vi "test Import-Export Custom Device.vi"(8 "error in":errorcluster, 11 "TestCase in":refnum<class "Scripting.lvclass">) -> (0 "error out":errorcluster, 3 "TestCase out":refnum<class "Scripting.lvclass">)   [LabVIEW 2020, in "Scripting.lvclass"]
uses:
  Scripting.lvclass
  C:/dev/git/niveristand-custom-device-testing-tools/VeriStandScriptingTestCase/VeriStandScriptingTestCase.lvclass
  niveristand-custom-device-testing-tools/VeriStandScriptingTestCase/VeriStandScriptingTestCase.lvclass/VeriStandScriptingTestCase.ctl
  NationalInstruments.VeriStand.SystemDefinitionAPI
  niveristand-custom-device-testing-tools/VeriStandScriptingTestCase/Read Target.vi
  Scripting/Custom Device/Import Custom Device (In Place).vi
  Scripting/Custom Device/Import Custom Device (New).vi
  Scripting/AIM MIL-STD-1553 Scripting.lvlib
  <vilib>/addons/_JKI Toolkits/VI Tester/TestCase.llb/TestCase.lvclass
  niveristand-custom-device-testing-tools/VeriStandTestUtilities/VeriStandTestUtilities.lvlib
  C:/Program Files (x86)/National Instruments/LabVIEW 2020/vi.lib/addons/_JKI Toolkits/VI Tester/TestCase.llb/TestCase.lvclass
  C:/dev/git/niveristand-aim-milStd1553-custom-device/Source/Custom Device Support/Tests/Unit/Scripting/Scripting.lvclass
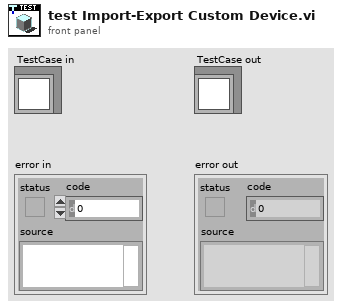
[diagram p1: front panel]
types:
  T1 = typedef "Custom Device API.lvlib/Custom Device Item Ref.ctl" = u64
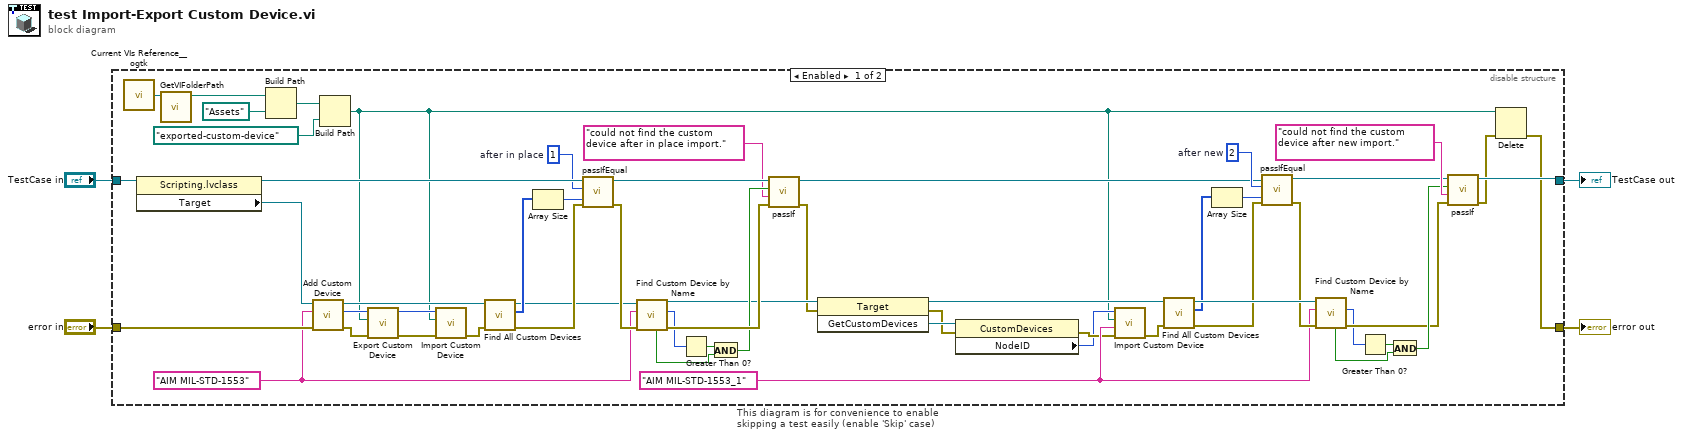
[diagram p0: block diagram]
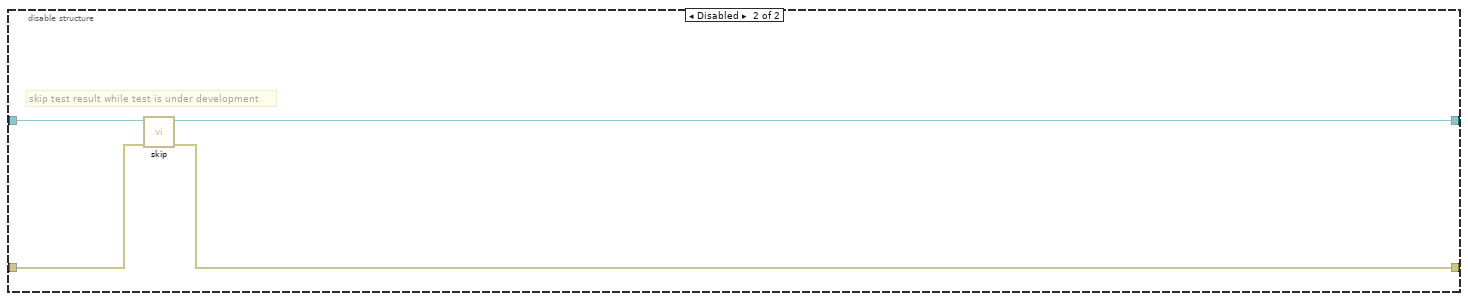
[diagram p2: hidden frame]
diagram:
  n1 = disable-structure "This diagram is for convenience to enable skipping a test easily (enable 'Skip' case)" shown="Enabled" {
    disable-tunnel: "TestCase in" -> [w59 w64]
    disable-tunnel: [w16 w62] -> w4
    disable-tunnel: [w5 w63] -> w2
    disable-tunnel: "error in" -> [w60 w61]
    frame Enabled {
      w17 = "AIM MIL-STD-1553_1" ("name")
      w22 = 2  # after new
      w43 = 1  # after in place
      w39 = "AIM MIL-STD-1553" ("name")
      n2 = call <userlib>:"Current VIs Reference__ogtk.vi"() -> ("Current VI's reference"=w52:refnum<vi>)  [unwired: 5 in]
      n3 = property class="Scripting.lvclass"(reference=w59) -> (reference out=w57:refnum<class "Scripting.lvclass">, "Target"=w58:refnum<k24>)  [unwired: 1 in, 1 out]
      n4 = call "GetVIFolderPath.vi"("VI Reference in"=w52) -> ("VI Folder Path out"=w51:path)  [unwired: 9 in, 1 out]
      n5 = Build Path(base path=w51, name or relative path=path "Assets") -> (appended path=w49:path)
      n6 = call "Add Custom Device.vi"("error in"=w60, "custom device name"=w39, "target"=w58) -> ("error out"=w54:errorcluster, "custom device"=w55:T1, "target out"=w47:refnum<k24>)  [unwired: 6 in]
      n7 = Build Path(base path=w49, name or relative path=path "exported-custom-device") -> (appended path=w7:path)
      n8 = call "Export Custom Device.vi"("error in"=w54, "path"=w7, "custom device"=w55) -> ("error out"=w53:errorcluster, "custom device out"=w56:T1)  [unwired: 7 in]
      n9 = call-poly "Import Custom Device.vi"("error in"=w53, "path"=w7, "custom device"=w56) -> ("error out"=w46:errorcluster)  [unwired: 7 in, 1 out]
      n10 = call "Find All Custom Devices.vi"("error in"=w46, "target"=w47) -> ("error out"=w42:errorcluster, "custom devices"=w45:T1[], "target out"=w40:refnum<k24>)  [unwired: 7 in]
      n11 = Array Size(array=w45) -> (size(s)=w44:i32)
      n12 = call-dynamic "passIfEqual.vi"("error in (no error)"=w42, "y"=w44, "x"=w43, "TestCase in"=w57) -> ("error out"=w41:errorcluster, "TestCase out"=w36:refnum<class "Scripting.lvclass">)  [unwired: 6 in]
      n13 = call "Find Custom Device by Name.vi"("error in"=w41, "custom device name"=w39, "target"=w40) -> ("error out"=w35:errorcluster, "custom device"=w15:T1, "target out"=w12:refnum<k24>, "found?"=w37:bool)  [unwired: 5 in]
      n14 = Greater Than 0?(x=w15) -> (x > 0?=w38:bool)
      n15 = And(x=w38, y=w37) -> (x .and. y?=w34:bool)
      n16 = call-dynamic "passIf.vi"("error in (no error)"=w35, "message (\"\")"="could not find the custom device after in place import." ("message (\"\")"), "pass"=w34, "TestCase in"=w36) -> ("error out"=w9:errorcluster, "TestCase out"=w18:refnum<class "Scripting.lvclass">)  [unwired: 6 in]
      n17 = invoke on="Invoke Node" class="Target" method="GetCustomDevices"(reference=w12, error in=w9) -> (reference out=w11:refnum<k24>, error out=w13:errorcluster, "GetCustomDevices"=w14:refnum<k24>)  [unwired: 1 in]
      n18 = property on="Property Node" class="CustomDevices"(reference=w14, error in=w13) -> (error out=w10:errorcluster, "NodeID"=w8:u64)  [unwired: 1 out]
      n19 = call-poly "Import Custom Device.vi"("error in"=w10, "name"=w17, "path"=w7, "custom devices"=w8) -> ("error out"=w19:errorcluster)  [unwired: 5 in, 2 out]
      n20 = call "Find All Custom Devices.vi"("error in"=w19, "target"=w11) -> ("error out"=w23:errorcluster, "custom devices"=w20:T1[], "target out"=w25:refnum<k24>)  [unwired: 7 in]
      n21 = Array Size(array=w20) -> (size(s)=w21:i32)
      n22 = call-dynamic "passIfEqual.vi"("error in (no error)"=w23, "y"=w21, "x"=w22, "TestCase in"=w18) -> ("error out"=w24:errorcluster, "TestCase out"=w29:refnum<class "Scripting.lvclass">)  [unwired: 6 in]
      n23 = call "Find Custom Device by Name.vi"("error in"=w24, "custom device name"=w17, "target"=w25) -> ("error out"=w30:errorcluster, "custom device"=w26:T1, "found?"=w28:bool)  [unwired: 5 in, 1 out]
      n24 = Greater Than 0?(x=w26) -> (x > 0?=w27:bool)
      n25 = And(x=w27, y=w28) -> (x .and. y?=w31:bool)
      n26 = call-dynamic "passIf.vi"("error in (no error)"=w30, "message (\"\")"="could not find the custom device after new import." ("message (\"\")"), "pass"=w31, "TestCase in"=w29) -> ("error out"=w6:errorcluster, "TestCase out"=w16:refnum<class "Scripting.lvclass">)  [unwired: 6 in]
      n27 = Delete(path (use dialog)=w7, error in=w6) -> (error out=w5:errorcluster)  [unwired: 3 in, 2 out]
    }
    frame Disabled {
      # "skip test result while test is under development"
      n28 = call <vilib>:"skip.vi"("error in (no error)"=w61, "TestCase in"=w64) -> ("error out"=w63:errorcluster, "TestCase out"=w62:refnum<class "Scripting.lvclass">)  [unwired: 8 in]
    }
  }
  "error out" <- w2
  "TestCase out" <- w4
